vi "Fit.vi"(8 "error in (no error)":errorcluster caption="entrée d'erreur (pas d'erreur)", 9 "y":string[][](array[string]), 10 "X":string[][](array[string]), 11 "IterativeImputer.lvclass":refnum<class "IterativeImputer.lvclass">) -> (0 "error out":errorcluster caption="sortie d'erreur", 2 "String Data":string, 3 "IterativeImputer.lvclass":refnum<class "IterativeImputer.lvclass">)   [LabVIEW 2020, in "IterativeImputer.lvclass"]
doc: "Fits the imputer on X and return self.\n\nReturns : \n\n- String : OK"
uses:
  IterativeImputer.lvclass
  IterativeImputer.lvclass/IterativeImputer.ctl
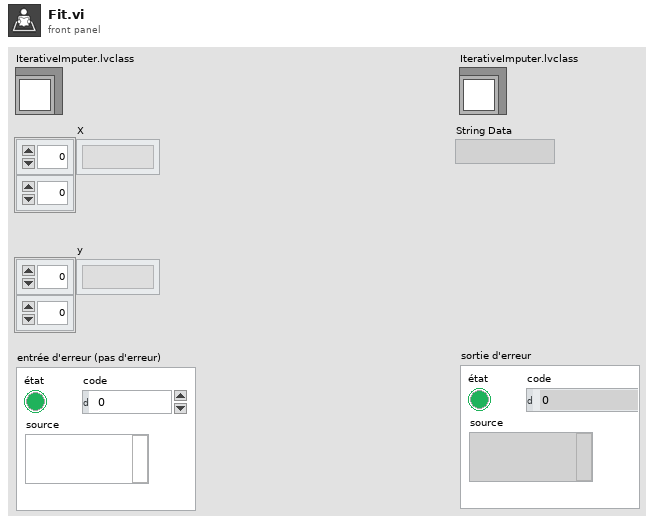
[diagram p1: front panel]
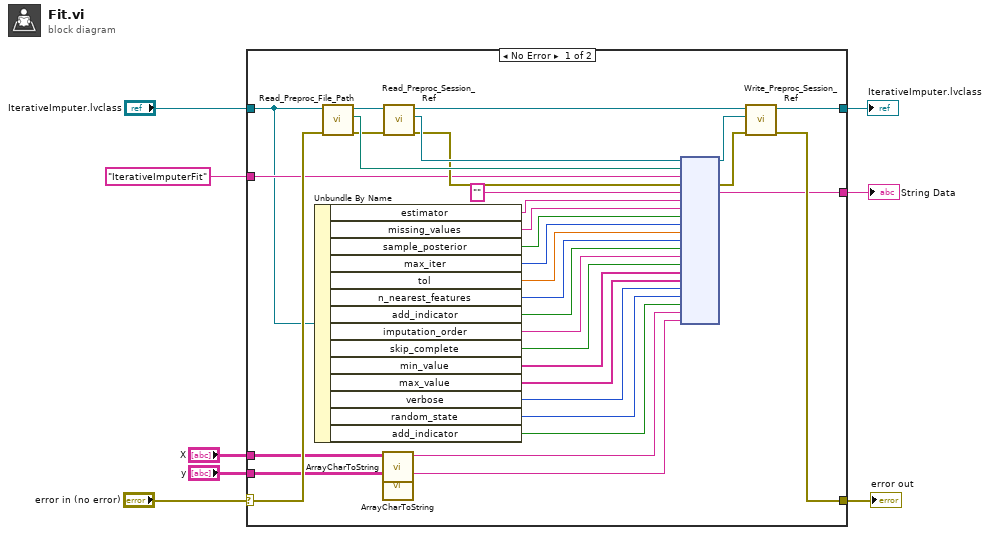
[diagram p0: block diagram]
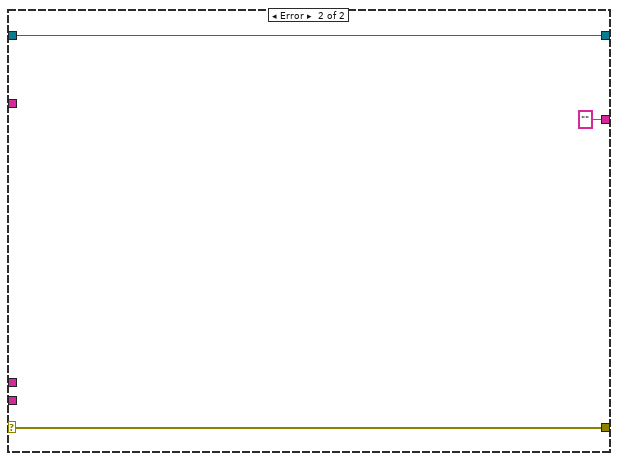
[diagram p2: hidden frame]
diagram:
  n1 = case shown="No Error" "error in (no error)" {
    selector: "error in (no error)" -> [w32 w44]
    tunnel: [w31 w44] -> w7
    tunnel: [w30 w43] -> w5
    tunnel: "IterativeImputer.lvclass" -> [w27 w43]
    tunnel: "IterativeImputerFit" ("Fonction") -> [w29 _]
    tunnel: [w28 ""] -> w3
    tunnel: "X" -> [w12 _]
    tunnel: "y" -> [w10 _]
    frame No Error {
      n2 = Unbundle By Name(w27) -> ("estimator"=w26:string, "missing_values"=w25:string, "sample_posterior"=w24:bool, "max_iter"=w23:i32, "tol"=w22:dbl, "n_nearest_features"=w21:i32, "add_indicator"=w20:bool, "imputation_order"=w19:string, "skip_complete"=w18:bool, "min_value"=w17:string[], "max_value"=w16:string[], "verbose"=w15:i32, "random_state"=w14:i32, "add_indicator"=w13:bool)
      n3 = call-dynamic "Read_Preproc_File_Path.vi"("error in (no error)"=w32, "Python in"=w27) -> ("error out"=w36:errorcluster, "File_Path"=w39:path, "Python out"=w41:refnum<class "IterativeImputer.lvclass">)  [unwired: 7 in]
      n4 = call "ArrayCharToString.vi"("TAB"=w12) -> ("Instruction"=w11:string)  [unwired: 10 in]
      n5 = call "ArrayCharToString.vi"("TAB"=w10) -> ("Instruction"=w9:string)  [unwired: 10 in]
      n6 = call-dynamic "Read_Preproc_Session_Ref.vi"("error in (no error)"=w36, "Python in"=w41) -> ("error out"=w37:errorcluster, "Session_ref"=w38:refnum<k35>, "Python out"=w40:refnum<class "IterativeImputer.lvclass">)  [unwired: 7 in]
      n7 = node(w38, w39, w29, w37, "", w26, w25, w24, w23, w22, w21, w20, w19, w18, w17, w16, w15, w14, w13, w11, w9) -> (w33:refnum<k35>, w35:errorcluster, w28:string)  [unwired: 16 in, 2 out]
      n8 = call-dynamic "Write_Preproc_Session_Ref.vi"("error in (no error)"=w35, "Session_ref"=w33, "Python in"=w40) -> ("error out"=w31:errorcluster, "Python out"=w30:refnum<class "IterativeImputer.lvclass">)  [unwired: 7 in]
    }
    frame Error {
    }
  }
  "error out" <- w7
  "IterativeImputer.lvclass" <- w5
  "String Data" <- w3
